vi "Write frames.vi"(8 "error in (no error)":errorcluster, 10 "frames":T1[](array[typedef]), 11 "database file in":refnum<class "database file.lvclass">) -> (0 "error out":errorcluster, 3 "database file out":refnum<class "database file.lvclass">)   [LabVIEW 2013, in "database file.lvclass"]
uses:
  database file.lvclass
  J1939 Library/Configuration/TypeDefs/J1939 db frame.ctl
  J1939 Library/Configuration/TypeDefs/J1939 db signal.ctl
  database file.lvclass/database file.ctl
  J1939 Library/J1939.lvlib
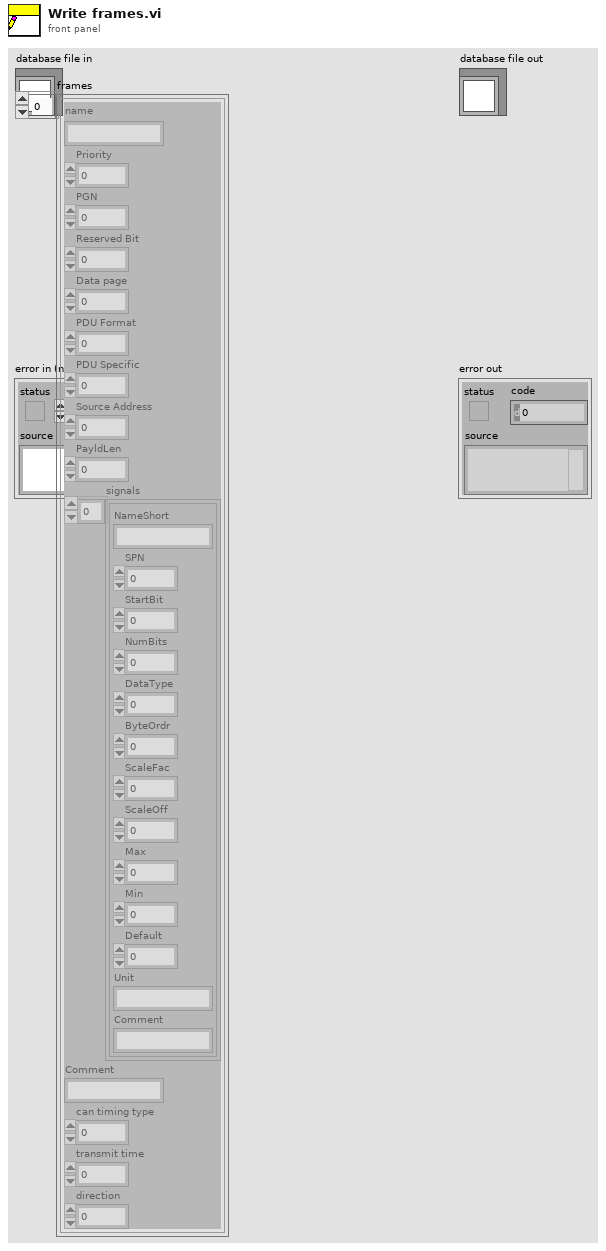
[diagram p1: front panel]
types:
  T1 = typedef "J1939.lvlib/J1939 db frame.ctl" = cluster{"name":string, "Priority":u8, "PGN":u32, "Reserved Bit":u8, "Data page":u8, "PDU Format":u8, "PDU Specific":u8, "Source Address":u8, "PayldLen":u32, "signals":T2[], "Comment":string, "can timing type":u32, "transmit time":dbl, "direction":u16}
  T2 = typedef "J1939.lvlib/J1939 db signal.ctl" = cluster{"NameShort":string, "SPN":i32, "StartBit":u32, "NumBits":u32, "DataType":u32, "ByteOrdr":u32, "ScaleFac":dbl, "ScaleOff":dbl, "Max":dbl, "Min":dbl, "Default":dbl, "Unit":string, "Comment":string}
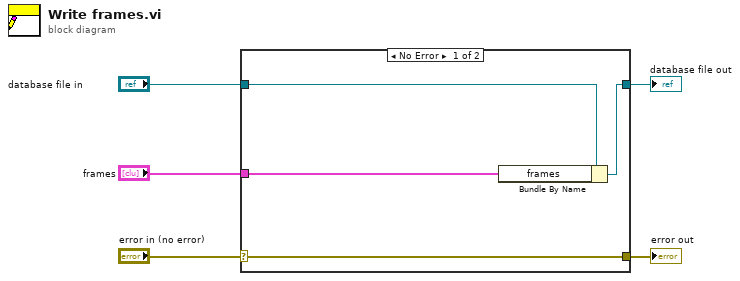
[diagram p0: block diagram]
diagram:
  n1 = case shown="No Error" "error in (no error)" {
    selector: "error in (no error)" -> [w9 w10]
    tunnel: [w9 w10] -> w4
    tunnel: [w7 w11] -> w2
    tunnel: "database file in" -> [w8 w11]
    tunnel: "frames" -> [w6 _]
    frame No Error {
      n2 = Bundle By Name(cluster=w8, "frames"=w6) -> (w7:refnum<class "database file.lvclass">)
    }
    frame Error {
    }
  }
  "error out" <- w4
  "database file out" <- w2
